vi "GetPrivateQueueMessage.vi"(8 "error in (no error)":errorcluster, 11 "DAQmx":refnum<class "DAQmx.lvclass">) -> (0 "error out":errorcluster, 1 "argument":string, 2 "command":T1, 3 "DAQmx out":refnum<class "DAQmx.lvclass">)   [LabVIEW 2019, in "DAQmx.lvclass"]
uses:
  DAQmx.lvclass
  typedefs/DAQmx.Commands--enum.ctl
  DAQmx.lvclass/DAQmx.ctl
  typedefs/Message--Cluster.ctl
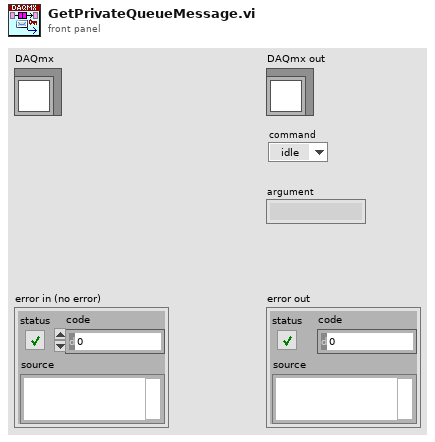
[diagram p1: front panel]
types:
  T1 = typedef "DAQmx.lvclass/DAQmx.Commands--enum.ctl" = enum16{"idle", "start", "stop", "calibrate", "auto", "exit"}
  T2 = typedef "DAQmx.lvclass/Message--Cluster.ctl" = cluster{"command":T1, "Argument":string}
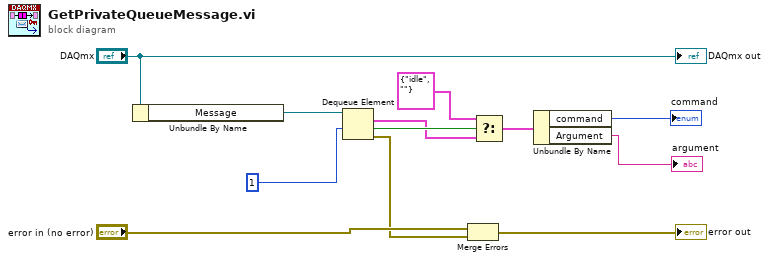
[diagram p0: block diagram]
diagram:
  n1 = Unbundle By Name("DAQmx") -> ("Message"=w12:refnum<queue>)
  n2 = Dequeue Element(queue=w12, timeout in ms (-1)=1) -> (element=w6:T2, timed out?=w11:bool, error out=w9:errorcluster)  [unwired: 1 in, 1 out]
  n3 = Merge Errors("error in (no error)", w9) -> (→"error out":errorcluster)
  n4 = Select(t=T2 {"command"=enum."idle", "Argument"=""}, s=w11, f=w6) -> (s? t:f=w5:T2)
  n5 = Unbundle By Name(w5) -> ("command"=→"command":T1, "Argument"=→"argument":string)
  "DAQmx out" <- "DAQmx"
